vi "Add Text Token.vi"(8 "Error In":errorcluster, 11 "Parser In":refnum<class "Parser.lvclass">) -> (0 "Error Out":errorcluster, 3 "Parser Out":refnum<class "Parser.lvclass">)   [LabVIEW 2018, in "Toolkit.lvlib" / "Parser.lvclass"]
uses:
  Parser.lvclass
  Parser.lvclass/Parser.ctl
  Tokens/Text/Text.lvclass
  D:/Users/cfield/Code/Field R&D Services/Mustache/trunk/src/Mustache/Public/Tokens/Public/Abstract/Abstract.lvclass
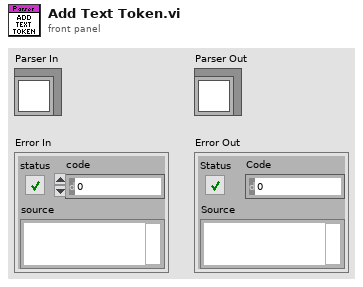
[diagram p1: front panel]
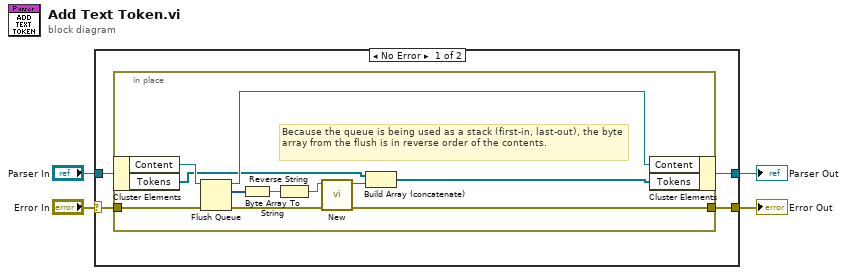
[diagram p0: block diagram]
diagram:
  n1 = case shown="No Error" "Error In" {
    selector: "Error In" -> [w5 w20]
    tunnel: [w8 w20] -> w4
    tunnel: [w7 w21] -> w3
    tunnel: "Parser In" -> [w6 w21]
    frame No Error {
      n2 = in-place {
        in-place-border: [w15] -> w8
        in-place-border: w5 -> [w11]
        # "Because the queue is being used as a stack (first-in, last-out), the byte array from the flush is in reverse order of the contents."
        n3 = in-place-cluster #1(w6) -> ("Content"=w19:refnum<queue>, "Tokens"=w14:refnum<class "Abstract.lvclass">[])
        n4 = Flush Queue(queue=w19, error in (no error)=w11) -> (queue out=w18:refnum<queue>, remaining elements=w17:u8[], error out=w16:errorcluster)
        n5 = Byte Array To String(unsigned byte array=w17) -> (string=w10:string)
        n6 = Reverse String(1:w10) -> (0:w9:string)
        n7 = call "New.vi"("Error In"=w16, "Content"=w9) -> ("Error Out"=w15:errorcluster, "Text"=w13:refnum<class "Text.lvclass">)  [unwired: 8 in]
        n8 = Build Array (concatenate)(w14, w13) -> (w12:refnum<class "Abstract.lvclass">[])
        n9 = in-place-cluster #1("Content"=w18, "Tokens"=w12) -> (w7:refnum<class "Parser.lvclass">)
      }
    }
    frame Error {
    }
  }
  "Error Out" <- w4
  "Parser Out" <- w3
